vi "Set Or Get Edit Position.vi"(8 "error in (no error)":errorcluster caption="错误输入（无错误）", 9 "Mode":T2, 10 "Edit Pos In":T1 caption="编辑位置", 11 "Table Ref In":refnum<vi>) -> (0 "error out":errorcluster caption="错误输出", 2 "Edit Pos Out":T1 caption="编辑位置", 3 "Table Ref Out":refnum<vi>)   [LabVIEW 2012, in "Table Tool.lvlib"]
uses:
  Table Tool.lvlib
  GetOrSet.ctl
  <vilib>/Utility/miscctls.llb/LVRowAndColumnTypeDef.ctl
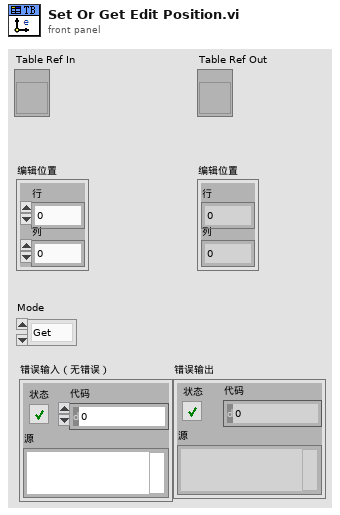
[diagram p1: front panel]
types:
  T1 = typedef "LVRowAndColumnTypeDef.ctl" = cluster{"Row":i32, "Column":i32}
  T2 = typedef "Table Tool.lvlib/GetOrSet.ctl" = enum16{"Get", "Set"}
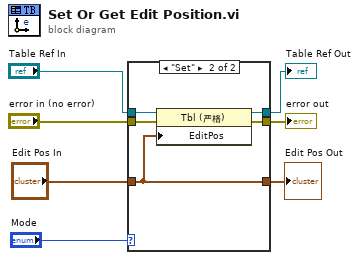
[diagram p0: block diagram]
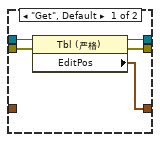
[diagram p2: hidden frame]
diagram:
  n1 = case shown="\"Set\"" "Mode" {
    tunnel: "Table Ref In" -> [w12 w17]
    tunnel: "error in (no error)" -> [w11 w16]
    tunnel: [w9 w15] -> w4
    tunnel: [w10 w14] -> w3
    tunnel: "Edit Pos In" -> [_ w13]
    tunnel: [w8 w13] -> w1
    frame "Get", Default {
      n2 = property class="Tbl (严格)"(reference=w12, error in=w11) -> (reference out=w10:refnum<vi>, error out=w9:errorcluster, "EditPos"=w8:T1)
    }
    frame "Set" {
      n3 = property class="Tbl (严格)"(reference=w17, error in=w16, "EditPos"=w13) -> (reference out=w14:refnum<vi>, error out=w15:errorcluster)
    }
  }
  "Table Ref Out" <- w3
  "error out" <- w4
  "Edit Pos Out" <- w1
